vi "Send File.vi"() -> ()   [LabVIEW 2017]
uses:
  State.ctl
  <vilib>/LVH/i3 JSON/JSON Parsing/Get Object Parameter Files/Get Object Parameter - Object.vi
  <vilib>/LVH/i3 JSON/JSON Parsing/Get Object Parameter Files/Get Object Parameter - Numeric.vi
  <vilib>/LVH/i3 JSON/i3-json.lvlib
panel:
  out "About":string="Simple app to send .cube3 files to Cube Printer.\nDeveloped by Luiz Renault. Feel free to send suggestions to luiz@luizrenault.com."
  in  "OK Button":bool
  out "Slide":u32(slide) max=3498616 scale=0.0..19143448.0
  out "error out":errorcluster
  out "Log:":string="Select File and Press Send."
  in  "file path (use dialog)":path=path "C:/Users/cadre/AppData/Local/Cubify/PrintFiles/testcube_10mm_1.cube3"
  out "Size":i32
  in  "address":string="192.168.1.100"
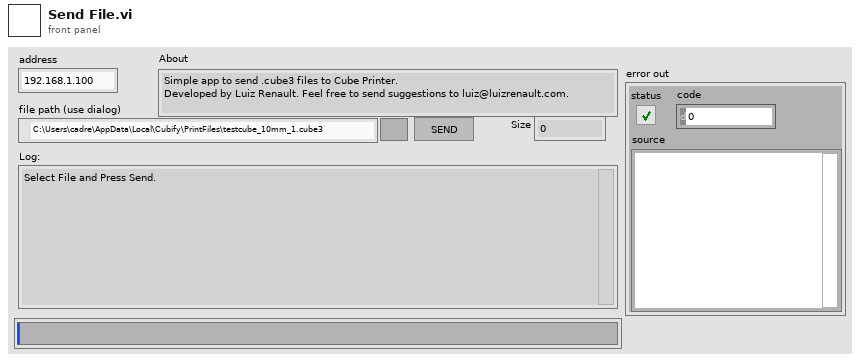
[diagram p1: front panel]
types:
  T1 = typedef "State.ctl" = enum16{"Pre Início", "Início", "Pronto Enviar", "Enviar Arquivo", "Esperar", "Imprimir", "Fim"}
  T2 = enum16{"Standard", "Buffered", "CRLF", "Immediate"}
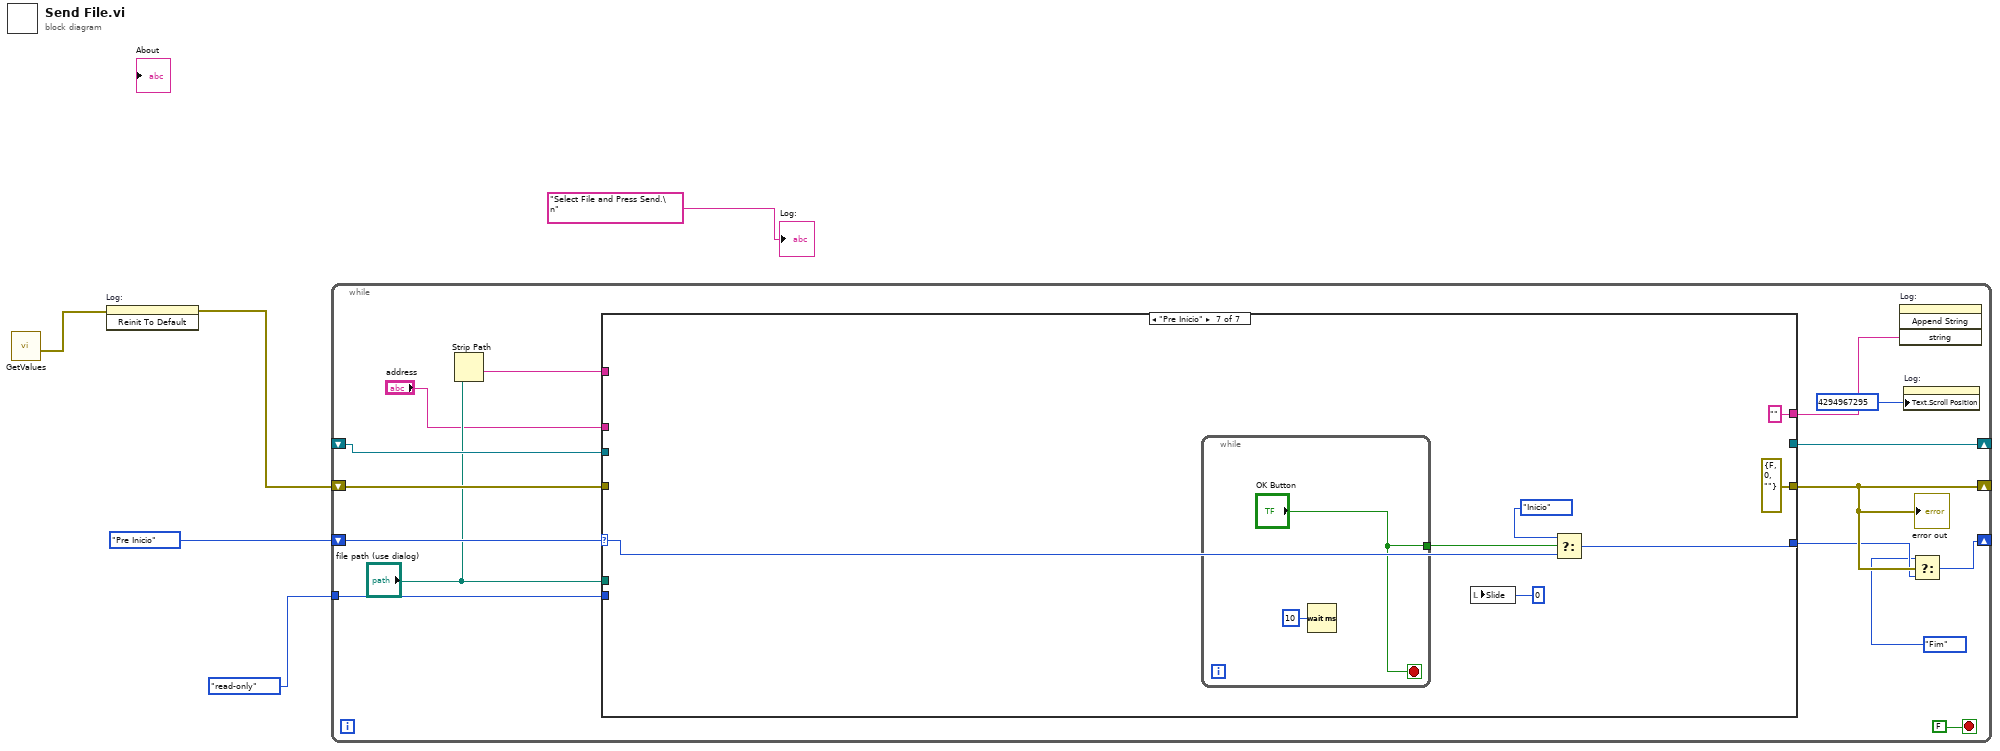
[diagram p0: block diagram]
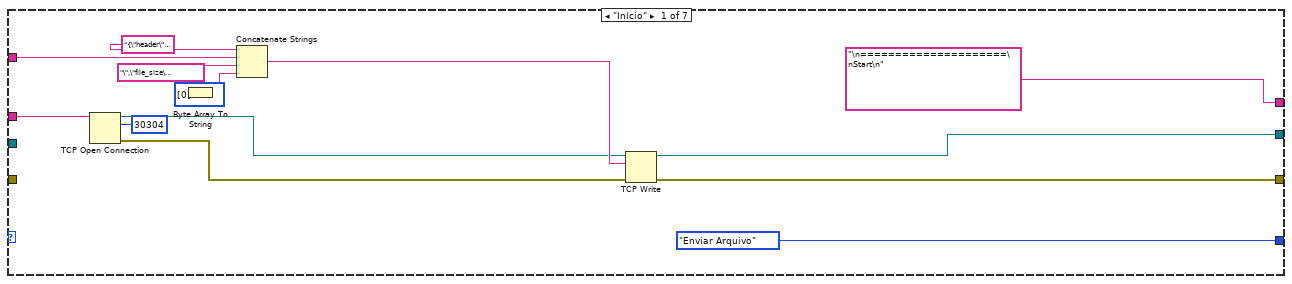
[diagram p2: hidden frame]
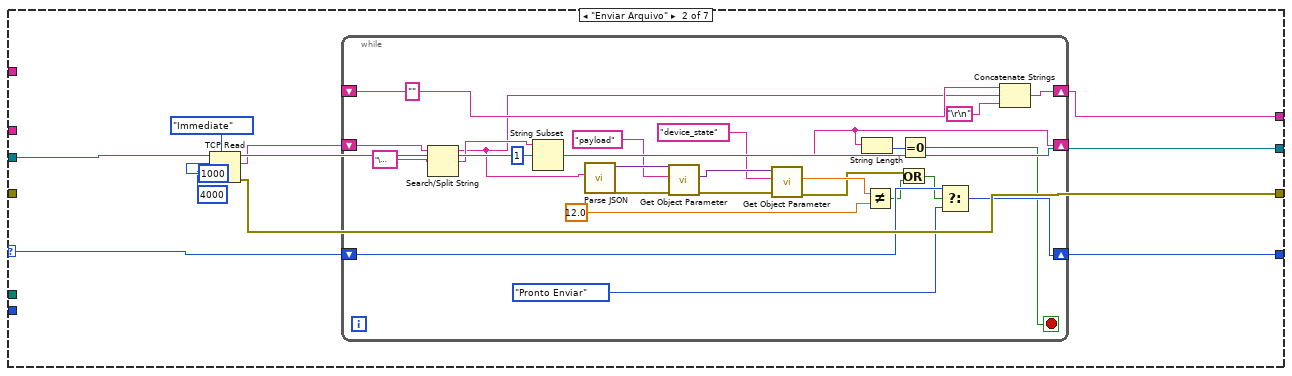
[diagram p3: hidden frame]
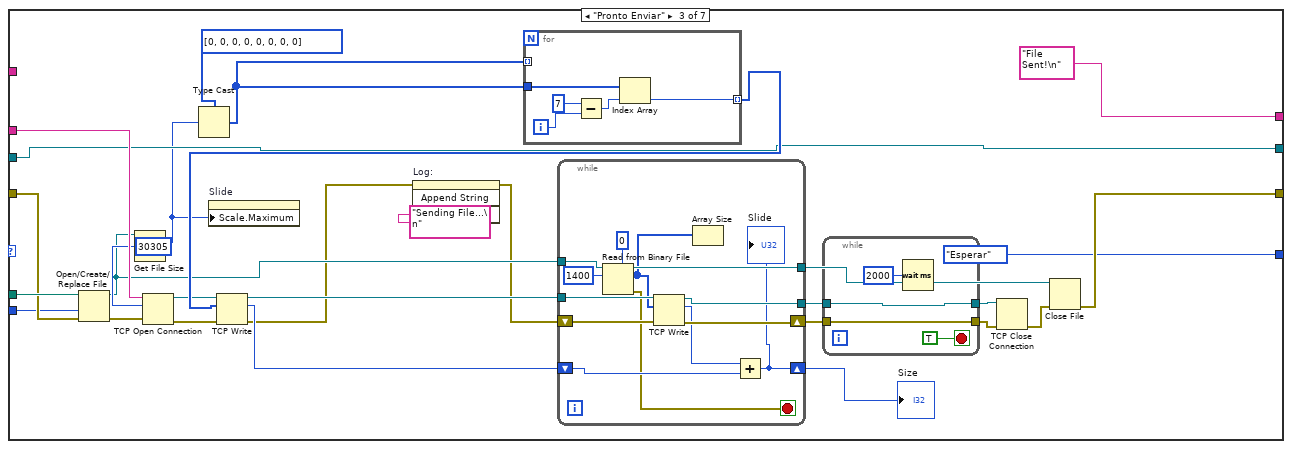
[diagram p4: hidden frame]
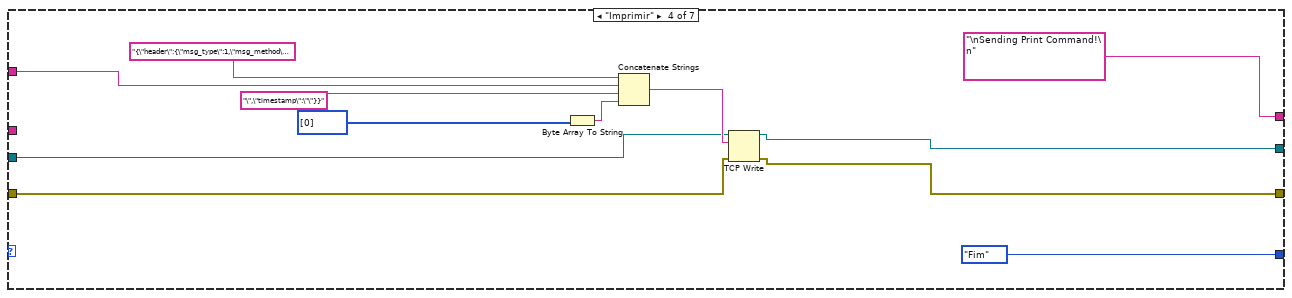
[diagram p5: hidden frame]
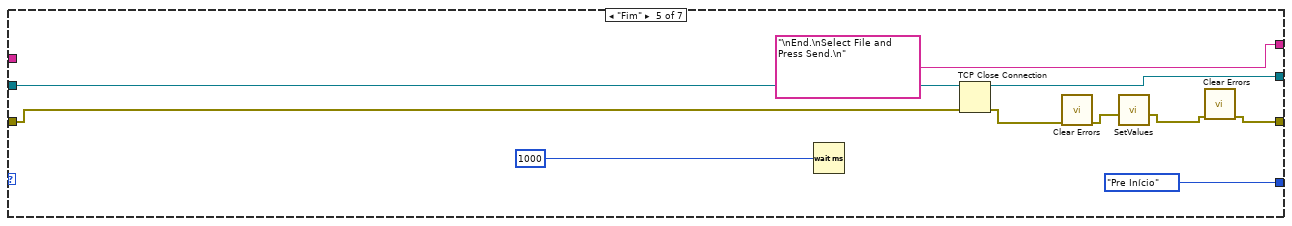
[diagram p6: hidden frame]
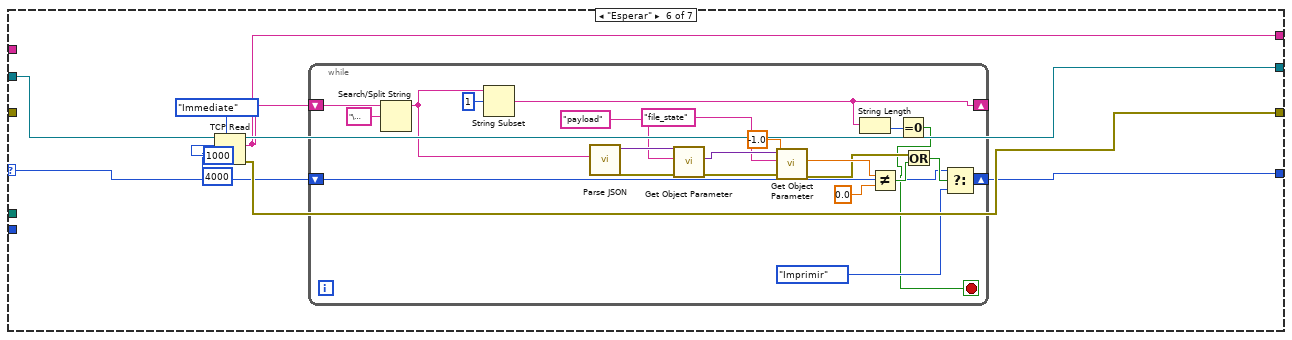
[diagram p7: hidden frame]
diagram:
  n1 = call "GetValues.vi"() -> ("error out"=w2:errorcluster)  [unwired: 11 in]
  n2 = invoke on="Log:" class="Str" method="Reinit To Default"(error in=w2) -> (error out=w1:errorcluster)  [unwired: 2 in, 2 out]
  n3 = while {
    shift-right: [w6] -> _
    shift-left: State."Pre Início" -> [w20]
    shift-right: [w13] -> _
    shift-left: _ -> [w19]
    shift-right: [w12] -> _
    shift-left: w1 -> [w18]
    tunnel: enum16{"read/write", "read-only", "write-only"}."read-only" ("access (0:read/write)") -> [w17]
    stop <- FALSE stop-if-true
    n4 = Strip Path(path="file path (use dialog)") -> (name=w16:string)  [unwired: 1 out]
    n5 = case shown="\"Pre Início\"" w20 {
      selector: w20 -> [_ w39 _ _ _ w145 w181]
      tunnel: "address" -> [w34 _ w80 _ _ _ _]
      tunnel: w16 -> [w31 _ _ w129 _ _ _]
      tunnel: [w26 w44 w75 w123 w139 w148 _] -> w13
      tunnel: [w25 w38 w78 w122 w134 w147 errorcluster {"status"=FALSE, "code"=0, "source"=""} ("error out")] -> w12
      tunnel: [State."Enviar Arquivo" w40 State."Esperar" State."Fim" State."Pre Início" w146 w180] -> w11
      tunnel: w19 -> [_ w45 w75 w127 w140 w149 _]
      tunnel: ["\n=====================\nStart\n" ("data out") w35 "File Sent!\n" ("data out") "\nSending Print Command!\n" ("data out") "\nEnd.\nSelect File and Press Send.\n" ("data out") w144 "" ("data out")] -> w8
      tunnel: w18 -> [_ _ w97 w126 w138 _ _]
      tunnel: "file path (use dialog)" -> [_ _ w98 _ _ _ _]
      tunnel: w17 -> [_ _ w96 _ _ _ _]
      frame "Início" {
        n6 = TCP Open Connection(address=w34, remote port or service name=u16 30304) -> (connection ID=w28:refnum<k5>, error out=w24:errorcluster)  [unwired: 3 in]
        n7 = Byte Array To String(unsigned byte array=u8[] [0]) -> (string=w22:string)
        n8 = Concatenate Strings("{\"header\":{\"msg_type\":1,\"msg_method\":102,\"version\":1},\"payload\":{\"file_name\":\"", w31, "\",\"file_size\":5.03435e+007}}", w22) -> (w29:string)
        n9 = TCP Write(connection ID=w28, data in=w29, error in (no error)=w24) -> (connection ID out=w26:refnum<k5>, error out=w25:errorcluster)  [unwired: 1 in, 1 out]
      }
      frame "Enviar Arquivo" {
        n10 = TCP Read(connection ID=w45, bytes to read=1000, 7:T2."Immediate" ("mode (standard)"), 9:4000 ("timeout ms (25000)")) -> (connection ID out=w44:refnum<k5>, data out=w37:string, error out=w38:errorcluster)  [unwired: 1 in]
        n11 = while {
          shift-right: [w62] -> w40
          shift-left: w39 -> [w61]
          shift-right: [w55] -> w35
          shift-left: "" -> [w56]
          shift-right: [w49] -> _
          shift-left: w37 -> [w53]
          stop <- w48 stop-if-true
          n12 = Search/Split String(string=w53, search string/char (-)="\u0000") -> (substring before match=w46:string, match + rest of string=w50:string)  [unwired: 1 in, 1 out]
          n13 = String Subset(string=w50, offset (0)=1) -> (substring=w49:string)  [unwired: 1 in]
          n14 = call <vilib>:"Parse JSON.vi"("JSON String"=w46) -> ("error out"=w68:errorcluster, "JSON Tree"=w70:variant)  [unwired: 7 in, 2 out]
          n15 = call-poly <vilib>:"Get Object Parameter.vi"("error in (no error)"=w68, "Parameter Name"="payload", "JSON Tree In (JSON Object)"=w70) -> ("error out"=w66:errorcluster, "JSON Object"=w67:variant)  [unwired: 5 in, 2 out]
          n16 = call-poly <vilib>:"Get Object Parameter.vi"("error in (no error)"=w66, "Parameter Name"="device_state", "JSON Tree In (JSON Object)"=w67) -> ("error out"=w60:errorcluster, "Double Value"=w64:dbl)  [unwired: 5 in, 2 out]
          n17 = String Length(string=w49) -> (length=w52:i32)
          n18 = Not Equal?(x=w64, y=12.0) -> (x != y?=w59:bool)
          n19 = Or(x=w60, y=w59) -> (x .or. y?=w58:bool)
          n20 = Equal To 0?(x=w52) -> (x = 0?=w48:bool)
          n21 = Select(t=w61, s=w58, f=State."Pronto Enviar") -> (s? t:f=w62:T1)
          n22 = Concatenate Strings(w56, w46, "\r\n") -> (w55:string)
        }
      }
      frame "Pronto Enviar" {
        n23 = Open/Create/Replace File(file path (use dialog)=w98, error in=w97, access (0:read/write)=w96) -> (refnum out=w76:refnum<file>, error out=w81:errorcluster)  [unwired: 3 in, 1 out]
        n24 = Get File Size(file=w76) -> (size (in bytes)=w74:i64)  [unwired: 1 in, 2 out]
        n25 = TCP Open Connection(address=w80, remote port or service name=u16 30305, error in (no error)=w81) -> (connection ID=w87:refnum<k5>, error out=w86:errorcluster)  [unwired: 2 in]
        n26 = Type Cast(type=u8[] [0, 0, 0, 0, 0, 0, 0, 0], x=w74) -> (*(type *) &x=w90:u8[])
        n27 = property on="Slide" class="Slide (strict)"("Scale.Maximum"=w74) -> ()  [unwired: 2 in, 2 out]
        n28 = for {
          tunnel: w90 -> [_] mode=indexing
          tunnel: w90 -> [w108]
          tunnel: [w104] -> w91 mode=indexing
          i -> [w106]
          n29 = Subtract(x=7, y=w106) -> (x-y=w107:i32)
          n30 = Index Array(array=w108, index=w107) -> (element=w104:u8)
        }
        n31 = TCP Write(connection ID=w87, data in=w91, error in (no error)=w86) -> (connection ID out=w88:refnum<k5>, bytes written=w89:i32, error out=w73:errorcluster)  [unwired: 1 in]
        n32 = invoke on="Log:" class="Str" method="Append String"(error in=w73, "string"="Sending File...\n") -> (error out=w72:errorcluster)  [unwired: 2 in, 3 out]
        n33 = while {
          tunnel: w88 -> [w121]
          shift-right: [w120] -> w92
          shift-left: w72 -> [w112]
          tunnel: [w119] -> w95
          shift-right: [w109] -> w83
          shift-left: w89 -> [w117]
          tunnel: [w114] -> w84
          tunnel: w76 -> [w110]
          stop <- w111 stop-if-true
          n34 = Read from Binary File(5:u8 0 ("data type"), 10:1400 ("count (1)"), 11:w110) -> (0:w111:errorcluster, 2:w113:u8[], 3:w114:refnum<file>)  [unwired: 3 in, 1 out]
          n35 = TCP Write(connection ID=w121, data in=w113, error in (no error)=w112) -> (connection ID out=w119:refnum<k5>, bytes written=w118:i32, error out=w120:errorcluster)  [unwired: 1 in]
          n36 = Array Size(array=w113) -> ()  [unwired: 1 out]
          n37 = Add(x=w118, y=w117) -> (x+y=w109:i32)
          "Slide" <- w109
        }
        "Size" <- w83
        n38 = while {
          tunnel: w92 -> [w103]
          tunnel: [w103] -> w93
          tunnel: [w102] -> w94
          tunnel: w95 -> [w102]
          stop <- TRUE stop-if-true
          n39 = Wait (ms)(milliseconds to wait=u32 2000) -> ()  [unwired: 1 out]
        }
        n40 = TCP Close Connection(connection ID=w94, error in (no error)=w93) -> (error out=w85:errorcluster)  [unwired: 1 in, 1 out]
        n41 = Close File(refnum=w84, error in=w85) -> (error out=w78:errorcluster)  [unwired: 1 out]
      }
      frame "Imprimir" {
        n42 = Byte Array To String(unsigned byte array=u8[] [0]) -> (string=w130:string)
        n43 = Concatenate Strings("{\"header\":{\"msg_type\":1,\"msg_method\":11,\"version\":1},\"payload\":{\"file_name\":\"", w129, "\",\"timestamp\":\"\"}}", w130) -> (w128:string)
        n44 = TCP Write(connection ID=w127, data in=w128, error in (no error)=w126) -> (connection ID out=w123:refnum<k5>, error out=w122:errorcluster)  [unwired: 1 in, 1 out]
      }
      frame "Fim" {
        n45 = Wait (ms)(milliseconds to wait=u32 1000) -> ()  [unwired: 1 out]
        n46 = TCP Close Connection(connection ID=w140, error in (no error)=w138) -> (connection ID out=w139:refnum<k5>, error out=w137:errorcluster)  [unwired: 1 in]
        n47 = call <vilib>:"Clear Errors.vi"("error in (no error)"=w137) -> ("error out"=w136:errorcluster)  [unwired: 5 in, 1 out]
        n48 = call "SetValues.vi"("error in"=w136) -> ("error out"=w135:errorcluster)  [unwired: 10 in]
        n49 = call <vilib>:"Clear Errors.vi"("error in (no error)"=w135) -> ("error out"=w134:errorcluster)  [unwired: 5 in, 1 out]
      }
      frame "Esperar" {
        n50 = TCP Read(connection ID=w149, bytes to read=1000, 7:T2."Immediate" ("mode (standard)"), 9:4000 ("timeout ms (25000)")) -> (connection ID out=w148:refnum<k5>, data out=w144:string, error out=w147:errorcluster)  [unwired: 1 in]
        n51 = while {
          shift-right: [w162] -> w146
          shift-left: w145 -> [w160]
          shift-right: [w155] -> _
          shift-left: w144 -> [w159]
          stop <- w153 stop-if-true
          n52 = Search/Split String(string=w159, search string/char (-)="\u0000") -> (substring before match=w157:string)  [unwired: 1 in, 2 out]
          n53 = String Subset(string=w157, offset (0)=1) -> (substring=w155:string)  [unwired: 1 in]
          n54 = call <vilib>:"Parse JSON.vi"("JSON String"=w157) -> ("error out"=w172:errorcluster, "JSON Tree"=w174:variant)  [unwired: 7 in, 2 out]
          n55 = call-poly <vilib>:"Get Object Parameter.vi"("error in (no error)"=w172, "Parameter Name"="payload", "JSON Tree In (JSON Object)"=w174) -> ("error out"=w170:errorcluster, "JSON Object"=w171:variant)  [unwired: 5 in, 2 out]
          n56 = call-poly <vilib>:"Get Object Parameter.vi"("error in (no error)"=w170, "Default Value if JSON Null"=-1.0, "Parameter Name"="file_state", "JSON Tree In (JSON Object)"=w171) -> ("error out"=w166:errorcluster, "Double Value"=w168:dbl)  [unwired: 4 in, 2 out]
          n57 = String Length(string=w155) -> (length=w154:i32)
          n58 = Not Equal?(x=w168, y=0.0) -> (x != y?=w165:bool)
          n59 = Equal To 0?(x=w154) -> (x = 0?=w153:bool)
          n60 = Or(x=w166, y=w165) -> (x .or. y?=w164:bool)
          n61 = Select(t=w160, s=w164, f=State."Imprimir") -> (s? t:f=w162:T1)
        }
      }
      frame "Pre Início" {
        n62 = while {
          tunnel: ["OK Button"] -> w179
          stop <- "OK Button" stop-if-true
          n63 = Wait (ms)(milliseconds to wait=u32 10) -> ()  [unwired: 1 out]
        }
        n64 = local write "Slide"(u32 0 ("Slide")) -> ()
        n65 = Select(t=State."Início", s=w179, f=w181) -> (s? t:f=w180:T1)
      }
    }
    "error out" <- w12
    n66 = invoke on="Log:" class="Str" method="Append String"("string"=w8) -> ()  [unwired: 3 in, 4 out]
    n67 = property on="Log:" class="Str"("Text.Scroll Position"=u32 4294967295) -> ()  [unwired: 2 in, 2 out]
    n68 = Select(t=State."Fim", s=w12, f=w11) -> (s? t:f=w6:T1)
  }
  "Log:" <- "Select File and Press Send.\n" ("Log:")
